vi "DN4_BfdCntr_PwModulatorWrite.vi"(8 "error in (no error)":errorcluster, 9 "pulse width(Array2D)":T1(array[cluster]), 10 "stop?":bool, 11 "Task ID":u32) -> (0 "error out":errorcluster, 2 "stopped":bool, 3 "Task out ID":u32)   [LabVIEW 2009]
uses:
  Windows/System32/AdvLvDaq.dll
panel:
  out "status":bool
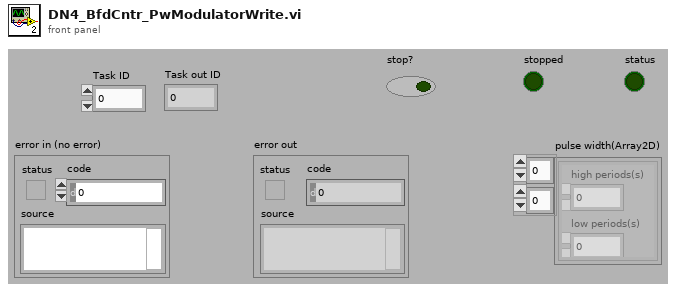
[diagram p1: front panel]
types:
  T1 = cluster{"high periods(s)":dbl, "low periods(s)":dbl}[][]
  T2 = cluster{"high periods(s)":dbl, "low periods(s)":dbl}[]
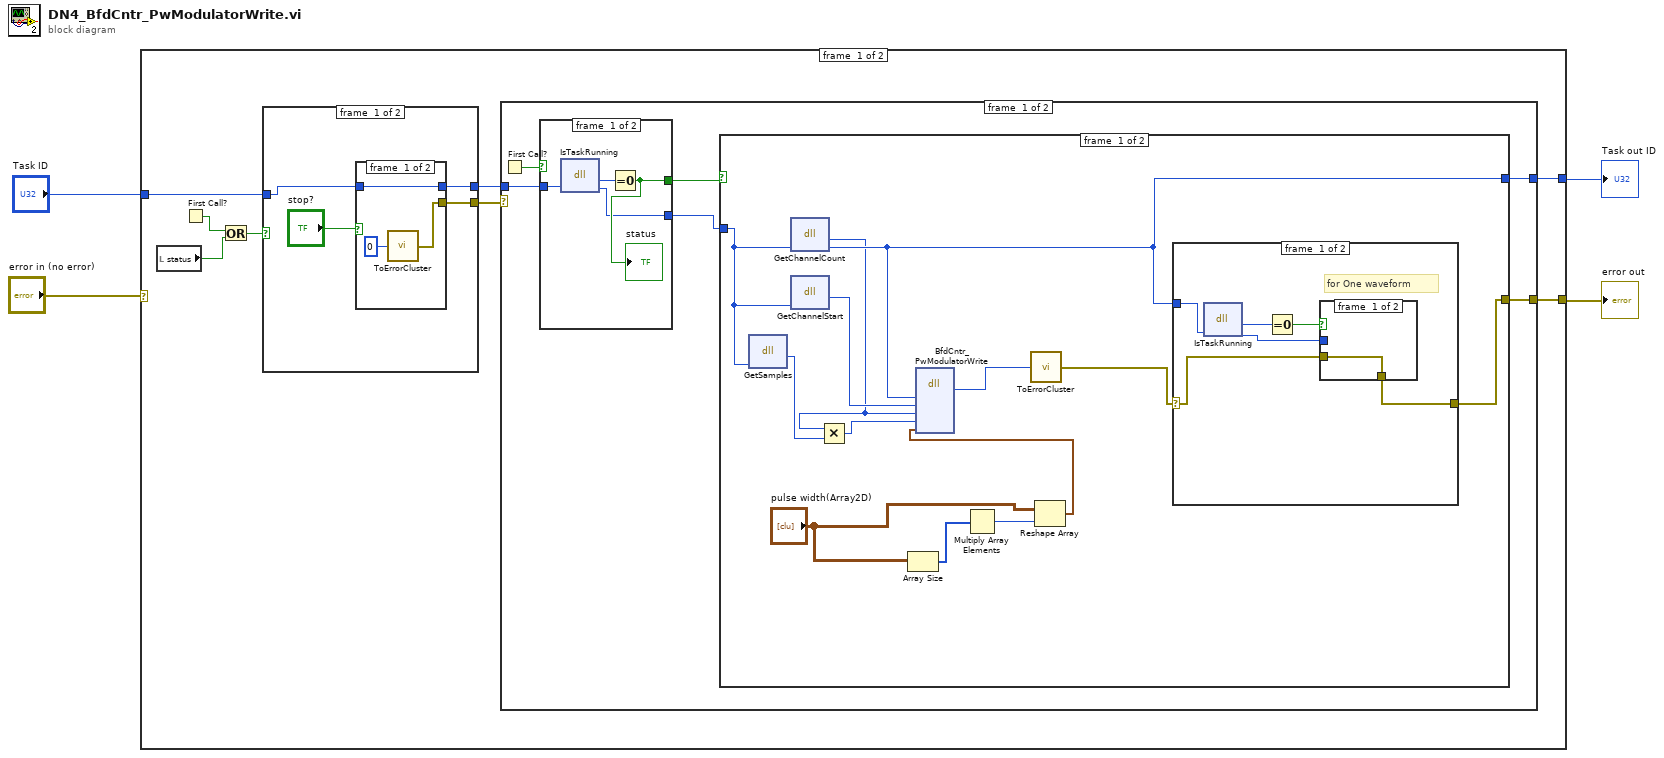
[diagram p0: block diagram]
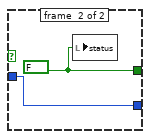
[diagram p2: hidden frame]
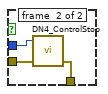
[diagram p3: hidden frame]
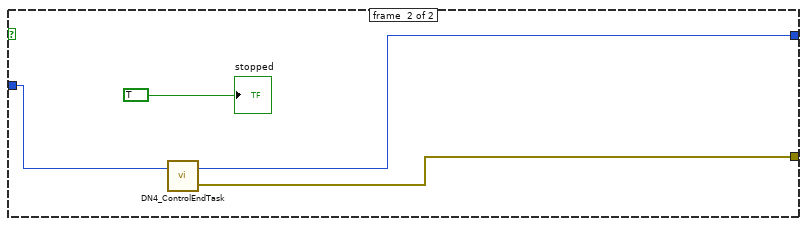
[diagram p5: hidden frame]
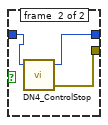
[diagram p7: hidden frame]
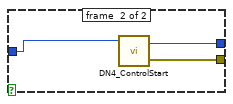
[diagram p8: hidden frame]
diagram:
  n1 = case shown="No Error" "error in (no error)" {
    selector: "error in (no error)" -> [_ w68]
    tunnel: "Task ID" -> [w9 w69]
    tunnel: [w6 w69] -> w2
    tunnel: [w5 w68] -> w1
    frame #0 {
      n2 = local read "status"() -> (w11:bool)
      n3 = First Call?() -> (First Call?: T/F=w12:bool)
      n4 = Or(x=w12, y=w11) -> (x .or. y?=w10:bool)
      n5 = case shown="False" w10 {
        tunnel: w9 -> [w55 w67]
        tunnel: [w57 w66] -> w7
        tunnel: [w56 w65] -> w8
        frame #0 {
          n6 = case shown="True" "stop?" {
            tunnel: [w60 w64] -> w57
            tunnel: [w61 w63] -> w56
            tunnel: w55 -> [w60 w62]
            frame #0 {
              n7 = call <userlib>:"ToErrorCluster.vi"("error code"=0) -> ("error out"=w61:errorcluster)
            }
            frame #1 {
              n8 = call <userlib>:"DN4_ControlStop.vi"("Task ID"=w62) -> ("error out"=w63:errorcluster, "Task ID"=w64:u32)  [unwired: 1 in, 2 out]
            }
          }
        }
        frame #1 {
          n9 = call <userlib>:"DN4_ControlStart.vi"("Task ID"=w67) -> ("error out"=w65:errorcluster, "Task ID"=w66:u32)  [unwired: 1 in, 1 out]
        }
      }
      n10 = case shown="No Error" w8 {
        selector: w8 -> [_ w53]
        tunnel: w7 -> [w15 w54]
        tunnel: [w18 w54] -> w6
        tunnel: [w17 w53] -> w5
        frame #0 {
          n11 = First Call?() -> (First Call?: T/F=w16:bool)
          n12 = case shown="False" w16 {
            tunnel: w15 -> [w21 w24]
            tunnel: [w20 w23] -> w14
            tunnel: [w19 w24] -> w13
            frame #0 {
              n13 = dll-call lib="C:/Windows/System32/AdvLvDaq.dll" fn="IsTaskRunning"("taskId"=w21) -> ("return type"=w22:i8, "taskId"=w19:u32)  [unwired: 3 in, 2 out]
              n14 = Equal To 0?(x=w22) -> (x = 0?=w20:bool)
              "status" <- w20
            }
            frame #1 {
              w23 = FALSE
              n15 = local write "status"(w23) -> ()
            }
          }
          n16 = case shown="False" w14 {
            tunnel: w13 -> [w37 w51]
            tunnel: [w34 w50] -> w18
            tunnel: [w36 w49] -> w17
            frame #0 {
              n17 = dll-call lib="C:/Windows/System32/AdvLvDaq.dll" fn="GetSamples"("taskId"=w37) -> ("return type"=w33:i32)  [unwired: 4 in, 2 out]
              n18 = dll-call lib="C:/Windows/System32/AdvLvDaq.dll" fn="GetChannelCount"("taskId"=w37) -> ("return type"=w29:i32, "taskId"=w34:u32)  [unwired: 3 in, 2 out]
              n19 = dll-call lib="C:/Windows/System32/AdvLvDaq.dll" fn="GetChannelStart"("taskId"=w37) -> ("return type"=w35:i32)  [unwired: 4 in, 2 out]
              n20 = Multiply(x=w29, y=w33) -> (x*y=w32:i32)
              n21 = Array Size(array="pulse width(Array2D)") -> (size(s)=w28:i32[])
              n22 = Multiply Array Elements(1:w28) -> (0:w27:i32)
              n23 = Reshape Array("pulse width(Array2D)", w27) -> (w25:T2)
              n24 = dll-call lib="C:/Windows/System32/AdvLvDaq.dll" fn="BfdCntr_PwModulatorWrite"("taskId"=w34, "cntrStart"=w35, "cntrCount"=w29, "count"=w32, "data"=w25) -> ("return type"=w31:i32)  [unwired: 8 in, 2 out]
              n25 = call <userlib>:"ToErrorCluster.vi"("error code"=w31) -> ("error out"=w30:errorcluster)
              n26 = case shown="No Error" w30 {
                selector: w30 -> [w38 w48]
                tunnel: w34 -> [w43 _]
                tunnel: [w39 w48] -> w36
                frame #0 {
                  # "for One waveform"
                  n27 = dll-call lib="C:/Windows/System32/AdvLvDaq.dll" fn="IsTaskRunning"("taskId"=w43) -> ("return type"=w42:i8, "taskId"=w40:u32)  [unwired: 3 in, 2 out]
                  n28 = Equal To 0?(x=w42) -> (x = 0?=w41:bool)
                  n29 = case shown="True" w41 {
                    tunnel: w40 -> [_ w47]
                    tunnel: [w44 w46] -> w39
                    tunnel: w38 -> [w44 w45]
                    frame #0 {
                    }
                    frame #1 {
                      n30 = call <userlib>:"DN4_ControlStop.vi"("error in (no error)"=w45, "Task ID"=w47) -> ("error out"=w46:errorcluster)  [unwired: 3 out]
                    }
                  }
                }
                frame #1 {
                }
              }
            }
            frame #1 {
              n31 = call <userlib>:"DN4_ControlEndTask.vi"("Task ID"=w51) -> ("error out"=w49:errorcluster, "Task ID"=w50:u32)  [unwired: 1 in]
              "stopped" <- TRUE
            }
          }
        }
        frame #1 {
        }
      }
    }
    frame #1 {
    }
  }
  "Task out ID" <- w2
  "error out" <- w1
